vi "Big or Little Endian.vi"(8 "error in":errorcluster, 11 "File":refnum<file>) -> (0 "error out":errorcluster, 2 "Litt/BigEnd":bool, 3 "File out":refnum<file>)   [LabVIEW 2013, in "Tiff reader.lvlib"]
doc: "Determines the byte order of the TIFF file."
uses:
  Tiff reader.lvlib
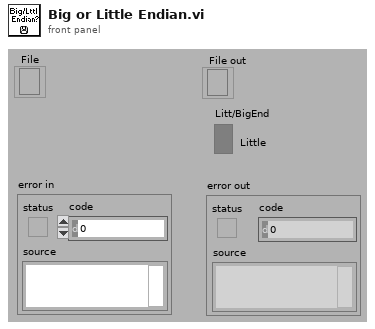
[diagram p1: front panel]
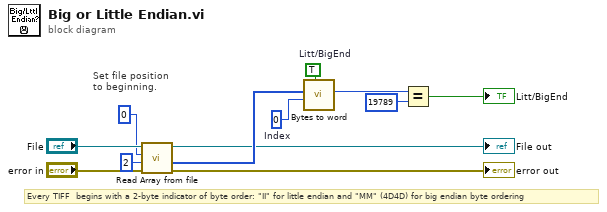
[diagram p0: block diagram]
diagram:
  w9 = TRUE  # Litt/BigEnd
  w12 = 0  # Index
  # "Every TIFF  begins with a 2-byte indicator of byte order: \"II\" for little endian and \"MM\" (4D4D) for big endian byte ordering"
  # "Set file position\nto beginning."
  n1 = call "Read Array from file.vi"("error in"="error in", "bytes to read"=2, "File location in"=i64 0, "File"="File") -> ("error out"=→"error out":errorcluster, "Array of U8s"=w4:u8[], "File out"=→"File out":refnum<file>)  [unwired: 1 out]
  n2 = call "Bytes to word.vi"("Litt/BigEnd"=w9, "Index"=w12, "Image Data in"=w4) -> ("Word"=w10:u16)  [unwired: 1 in, 5 out]
  n3 = Equal?(x=w10, y=u16 19789) -> (x = y?=→"Litt/BigEnd":bool)
